vi "PH_VacuumControl.set GUI elements.vi"(0 "i ref in":refnum<vi>, 5 "error in (no error)":errorcluster) -> (14 "i ref out":refnum<vi>, 19 "error out":errorcluster)   [LabVIEW 2014, in "PH_VacuumControl.lvlib"]
doc: "This VI manipulates GUI elements."
uses:
  PH_VacuumControl.lvlib
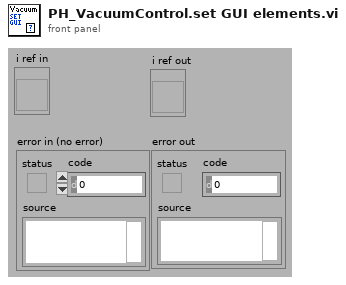
[diagram p1: front panel]
types:
  T1 = typedef "PH_VacuumControl.lvlib/PH_VacuumControl.i attribute.ctl" = cluster{"GUI Refs":cluster{"Exit":refnum<vi>, "Set Unit":refnum<vi>, "Device found":refnum<vi>, "Busy":refnum<vi>, "State":refnum<vi>, "Delete":refnum<vi>, "Channels":refnum<vi>, "Channel Name":refnum<vi>, "Trend":refnum<vi>, "Logarithmic":refnum<vi>, "Limit reached":refnum<vi>, "Channel Name 1 MT":refnum<vi>, "Channel Name 2 MT":refnum<vi>, "Trend MT":refnum<vi>, "Logarithmic MT":refnum<vi>, "Limit reached MT":refnum<vi>}, "Device found":bool, "Busy":bool, "Selected Unit":i32, "Channels [mbar]":T2, "Channel Names":cluster{"Channel 1":string, "Channel 2":string, "Channel 3":string, "Channel 4":string, "Channel 5":string, "Channel 6":string}, "Status":T3, "AGCxxx VISA Cluster":T4, "Instr Firmware Revision":string, "Service IDs Pressure":cluster{"Channel 1":i32, "Channel 2":i32, "Channel 3":i32, "Channel 4":i32, "Channel 5":i32, "Channel 6":i32}, "Service IDs Limits":cluster{"Channel 1":i32, "Channel 2":i32, "Channel 3":i32, "Channel 4":i32, "Channel 5":i32, "Channel 6":i32}, "Trend":cluster{"Start Point":timestamp, "Pressures [mbar] Channel 1":dbl[], "Pressures [mbar] Channel 2":dbl[], "Pressures [mbar] Channel 3":dbl[], "Pressures [mbar] Channel 4":dbl[], "Pressures [mbar] Channel 5":dbl[], "Pressures [mbar] Channel 6":dbl[], "Timebase [s]":i32[], "Trend Channel":u16, "Start Fit":dbl, "Trend Channel 1 MT":u16, "Trend Channel 2 MT":u16, "Start or continue Fit MT":dbl, "Continue or start Fit MT":dbl, "Datasets strored":i32, "Dataarray Size":i32}, "Running":bool}
  T2 = typedef "PH_VacuumControl.lvlib/PH_VacuumControl.Channels.ctl" = cluster{"Channel 1":dbl, "Channel 2":dbl, "Channel 3":dbl, "Channel 4":dbl, "Channel 5":dbl, "Channel 6":dbl, "Name Channel 1":string, "Name Channel 2":string, "Name Channel 3":string, "Name Channel 4":string, "Name Channel 5":string, "Name Channel 6":string, "Upper Limit":dbl, "Upper Limit 2":dbl, "Upper Limit 3":dbl, "Upper Limit 4":dbl, "Upper Limit 5":dbl, "Upper Limit 6":dbl}
  T3 = typedef "PH_StatusHandler.lvlib/PH_StatusHandler.Status.ctl" = i16
  T4 = typedef "AGCxxx - Driver.lvlib/AGCxxx VISA Control.ctl" = cluster{"VISA resource name":refnum<visa-resource-name>, "VISA Timeout Value (1000 ms)":u32, "Lock Timeout (1000 ms)":u32, "MAX Channel (6)":i32}
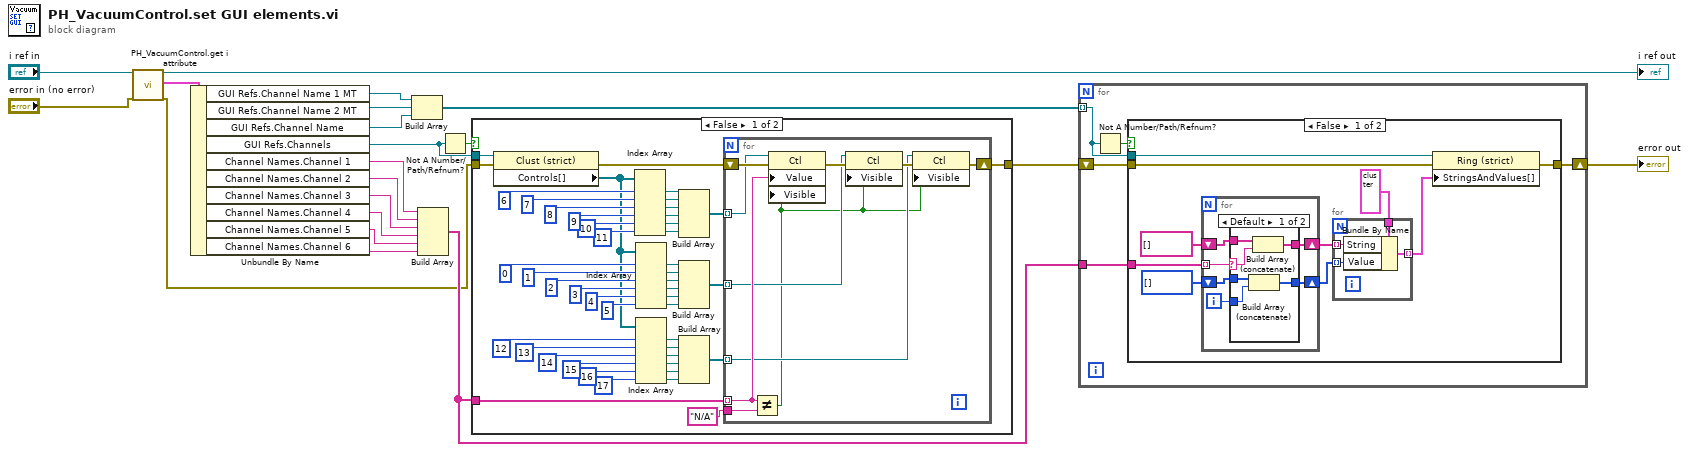
[diagram p0: block diagram]
diagram:
  n1 = call "PH_VacuumControl.get i attribute.vi"("i ref in"="i ref in", "error in (no error)"="error in (no error)") -> ("i ref out"=→"i ref out":refnum<vi>, "i attribute"=w19:T1, "error out"=w5:errorcluster)  [unwired: 15 in]
  n2 = Unbundle By Name(w19) -> ("GUI Refs.Channel Name 1 MT"=w3:refnum<vi>, "GUI Refs.Channel Name 2 MT"=w2:refnum<vi>, "GUI Refs.Channel Name"=w6:refnum<vi>, "GUI Refs.Channels"=w17:refnum<vi>, "Channel Names.Channel 1"=w15:string, "Channel Names.Channel 2"=w14:string, "Channel Names.Channel 3"=w13:string, "Channel Names.Channel 4"=w12:string, "Channel Names.Channel 5"=w11:string, "Channel Names.Channel 6"=w10:string)
  n3 = Build Array(w3, w2, w6) -> (w4:refnum<vi>[])
  n4 = Build Array(w15, w14, w13, w12, w11, w10) -> (w7:string[])
  n5 = Not A Number/Path/Refnum?(number/path/refnum=w17) -> (NaN/Path/Refnum?=w18:bool)
  n6 = case shown="False" w18 {
    tunnel: w17 -> [w66 _]
    tunnel: w5 -> [w65 w77]
    tunnel: [w51 w77] -> w8
    tunnel: w7 -> [w21 _]
    frame False {
      n7 = property class="Clust (strict)"(reference=w66, error in=w65) -> (error out=w52:errorcluster, "Controls[]"=w23:refnum<vi>[])  [unwired: 1 out]
      n8 = Index Array(array=w23, index #1=6 ("index"), index #2=7 ("index"), index #3=8 ("index"), index #4=9 ("index"), index #5=10 ("index"), index #6=11 ("index")) -> (element #1=w50:refnum<vi>, element #2=w49:refnum<vi>, element #3=w48:refnum<vi>, element #4=w47:refnum<vi>, element #5=w46:refnum<vi>, element #6=w45:refnum<vi>)
      n9 = Index Array(array=w23, index #1=0 ("index"), index #2=1 ("index"), index #3=2 ("index"), index #4=3 ("index"), index #5=4 ("index"), index #6=5 ("index")) -> (element #1=w44:refnum<vi>, element #2=w43:refnum<vi>, element #3=w42:refnum<vi>, element #4=w41:refnum<vi>, element #5=w40:refnum<vi>, element #6=w39:refnum<vi>)
      n10 = Index Array(array=w23, index #1=12 ("index"), index #2=13 ("index"), index #3=14 ("index"), index #4=15 ("index"), index #5=16 ("index"), index #6=17 ("index")) -> (element #1=w29:refnum<vi>, element #2=w28:refnum<vi>, element #3=w27:refnum<vi>, element #4=w26:refnum<vi>, element #5=w25:refnum<vi>, element #6=w24:refnum<vi>)
      n11 = Build Array(w50, w49, w48, w47, w46, w45) -> (w38:refnum<vi>[])
      n12 = Build Array(w44, w43, w42, w41, w40, w39) -> (w36:refnum<vi>[])
      n13 = Build Array(w29, w28, w27, w26, w25, w24) -> (w22:refnum<vi>[])
      n14 = for {
        shift-right: [w71] -> w51
        shift-left: w52 -> [w76]
        tunnel: w38 -> [w75] mode=indexing
        tunnel: w21 -> [w74] mode=indexing
        tunnel: "N/A" ("y") -> [w73]
        tunnel: w36 -> [w69] mode=indexing
        tunnel: w22 -> [w68] mode=indexing
        n15 = Not Equal?(x=w74, y=w73) -> (x != y?=w67:bool)
        n16 = property class="Ctl"(reference=w75, error in=w76, "Value"=w74, "Visible"=w67) -> (error out=w70:errorcluster)  [unwired: 1 out]
        n17 = property class="Ctl"(reference=w69, error in=w70, "Visible"=w67) -> (error out=w72:errorcluster)  [unwired: 1 out]
        n18 = property class="Ctl"(reference=w68, error in=w72, "Visible"=w67) -> (error out=w71:errorcluster)  [unwired: 1 out]
      }
    }
    frame True {
    }
  }
  n19 = for {
    tunnel: w7 -> [w80]
    tunnel: w4 -> [w79] mode=indexing
    shift-right: [w82] -> w9
    shift-left: w8 -> [w81]
    n20 = Not A Number/Path/Refnum?(number/path/refnum=w79) -> (NaN/Path/Refnum?=w78:bool)
    n21 = case shown="False" w78 {
      tunnel: [w92 w111] -> w82
      tunnel: w81 -> [w91 w111]
      tunnel: w80 -> [w87 _]
      tunnel: w79 -> [w85 _]
      frame False {
        n22 = for {
          tunnel: w87 -> [w98] mode=indexing
          shift-right: [w97] -> w90
          shift-left: string[] [] -> [w96]
          shift-right: [w95] -> w89
          shift-left: i32[] [] -> [w93]
          i -> [w94]
          n23 = case shown="Default" w98 {
            selector: w98 -> [w104 _]
            tunnel: [w103 w106] -> w97
            tunnel: w96 -> [w102 w106]
            tunnel: [w101 w105] -> w95
            tunnel: w94 -> [w100 _]
            tunnel: w93 -> [w99 w105]
            frame Default {
              n24 = Build Array (concatenate)(w99, w100) -> (w101:i32[])
              n25 = Build Array (concatenate)(w102, w104) -> (w103:string[])
            }
            frame "", "N/A" {
            }
          }
        }
        n26 = for {
          tunnel: [w110] -> w86 mode=indexing
          tunnel: cluster{"String":string, "Value":ext} {"String"="", "Value"=0.0} -> [w109]
          tunnel: w90 -> [w108] mode=indexing
          tunnel: w89 -> [w107] mode=indexing
          n27 = Bundle By Name(cluster=w109, "String"=w108, "Value"=w107) -> (w110:cluster{"String":string, "Value":ext})
        }
        n28 = property class="Ring (strict)"(reference=w85, error in=w91, "StringsAndValues[]"=w86) -> (error out=w92:errorcluster)  [unwired: 1 out]
      }
      frame True {
      }
    }
  }
  "error out" <- w9
